vi "Autonomous Independent.vi"() -> ()   [LabVIEW 2016]
doc: "This VI is called when autonomous begins, and will automatically be terminated when autonomous ends. You can carry out timed or sensor driven robot movement independently without needing to return to the caller."
uses:
  <vilib>/Rock Robotics/WPI/Utilities/WPI_GetSetVariantRefNum.vi
  <vilib>/Rock Robotics/Network Tables/NT Read String.vi
  <vilib>/Rock Robotics/Network Tables/NT Write Numeric Array.vi
  <vilib>/Rock Robotics/WPI/RobotDrive/WPI_RobotDriveArcadeDrive_Standard(NoSaturation).vi
panel:
  in  "PID":T1
  out "Sensor2Pos":dbl
  out "Sensor1Pos":dbl
  in  "Rotational Target":dbl
  out "SensorPos 2":dbl
  out "SensorPos":dbl
  in  "Target":dbl
  out "Current Movement, for debugging":T2 {"Y Joystick Value" scale=1.0..-1.0; "X Joystick Value" scale=-1.0..1.0}
  in  "Array of robot movements":T3(array[cluster])=[{"X Joystick Value"=0.39393939393939403, "Y Joystick Value"=0.0, "Delay (sec)"=1.0, "Movement Name"="turn"}, {"X Joystick Value"=-0.3737373737373737, "Y Joystick Value"=0.0, "Delay (sec)"=1.0, "Movement Name"="turn back"}] {"Y Joystick Value" scale=1.0..-1.0; "X Joystick Value" scale=-1.0..1.0}
  # "Be sure to right-click and choose Data Operations>>Make Current Value default if you want to save the array values with the VI"
  # "Position Closed Loop"
  # "Positive=Clockwise"
  # "Rotate"
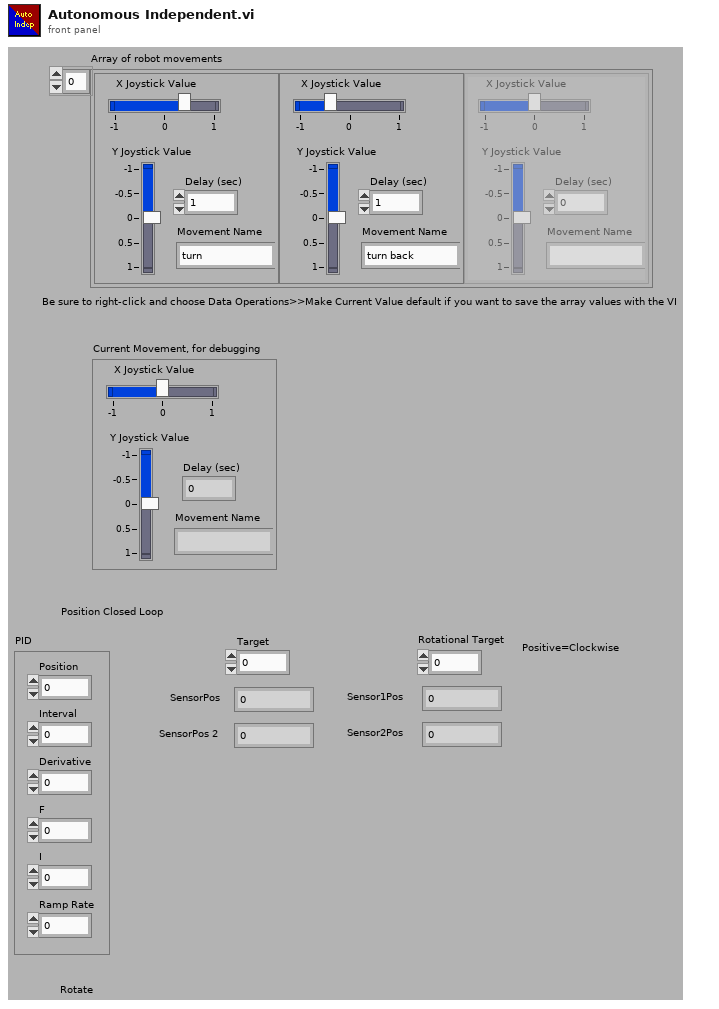
[diagram p1: front panel]
types:
  T1 = cluster{"Position":dbl, "Interval":dbl, "Derivative":dbl, "F":dbl, "I":dbl, "Ramp Rate":dbl}
  T2 = cluster{"X Joystick Value":dbl, "Y Joystick Value":dbl, "Delay (sec)":dbl, "Movement Name":string}
  T3 = cluster{"X Joystick Value":dbl, "Y Joystick Value":dbl, "Delay (sec)":dbl, "Movement Name":string}[]
  T4 = typedef "WPI_JoystickDevRef.ctl" = cluster{"Device":T5}
  T5 = typedef "WPI_JoystickDeviceEnum.ctl" = enum16{"USB 0", "USB 1", "USB 2", "USB 3", "USB 4", "USB 5"}
  T6 = typedef "WPI_RobotDriveDevRef.ctl" = cluster{"DevStatus":errorcluster, "Motors[]":T7[], "Square Inputs":bool, "Max Output":dbl}
  T7 = typedef "WPI_MotorControlDeviceRef.ctl" = cluster{"DeviceStatus":errorcluster, "Type":T8, "PWM":cluster{"PWM Channel":T9, "DeadBand":T10}, "CAN":cluster{"Device Number":u8, "SetOutput VI Ref":variant, "GetOutput VI Ref":variant, "Enable VI Ref":variant, "Disable VI Ref":variant, "Data":variant}, "Invert":bool}
  T8 = typedef "WPI_MotorControlType.ctl" = enum16{"PWM", "CAN"}
  T9 = typedef "FPGA_DIOPWMChannel.ctl" = enum8{"PWM 0", "PWM 1", "PWM 2", "PWM 3", "PWM 4", "PWM 5", "PWM 6", "PWM 7", "PWM 8", "PWM 9", "PWM MXP 0", "PWM MXP 1", "PWM MXP 2", "PWM MXP 3", "PWM MXP 4", "PWM MXP 5", "PWM MXP 6", "PWM MXP 7", "PWM MXP 8", "PWM MXP 9", "Invalid"}
  T10 = typedef "WPI_PWMDeadband.ctl" = cluster{"Name":string, "maxPositivePwm":i32, "minPositivePwm":i32, "centerPwm":i32, "maxNegativePwm":i32, "minNegativePwm":i32, "angularRange":u16}
  T11 = typedef "WPI_CANTalonSRX_GlobalStatus.ctl" = cluster{"Applied Throttle":dbl, "Module Enabled":bool, "CAN Error":errorcluster, "Closed Loop Error":dbl, "Forward Limit Switch Closed":bool, "Reverse Limit Switch Closed":bool, "Sensor Position":dbl, "Sensor Velocity":dbl, "Current":dbl, "Sticky Fault - Over Temp":bool, "Sticky Fault - Under Voltage":bool, "Sticky Fault - Forward Limit":bool, "Sticky Fault - Reverse Limit":bool, "Sticky Fault - Forward Soft Limit":bool, "Sticky Fault - Reverse Soft Limit":bool, "Brake is Enabled":bool, "Encoder Position":dbl, "Encoder Velocity":dbl, "Encoder Index Count":dbl, "Encoder A Pin State":bool, "Encoder B Pin State":bool, "Encoder Index Pin State":bool, "Analog In":dbl, "Analog In Velocity":dbl, "Temperature (C)":dbl, "Battery Voltage":dbl, "Control 5 Is Supported":bool, "Current Profile Slot Select":dbl, "Pos Div 8":bool, "Vel Div 4":bool, "Pulse Width Position":i32, "Pulse Width Velocity":i32, "Pulse Width Rise To Rise (us)":i32, "Pulse Width Rise To Fall (us)":i32, "Mot Prof Active Is Under Run":bool, "Mot Prof Active Has Under Run":bool, "Mot Prof Active Is Last":bool, "Mot Prof Active Velocity Only":bool, "Mot Prof Active Is Valid":bool, "Mot Prof Buffer Is Full":bool, "Mot Prof Active Profile Slot Select":i32, "Mot Prof NextID":i32, "Mot Prof Count":i32, "Mot Prof Active Velocity":dbl, "Mot Prof Active Position":dbl, "Mot Prof Output Enable":i32}
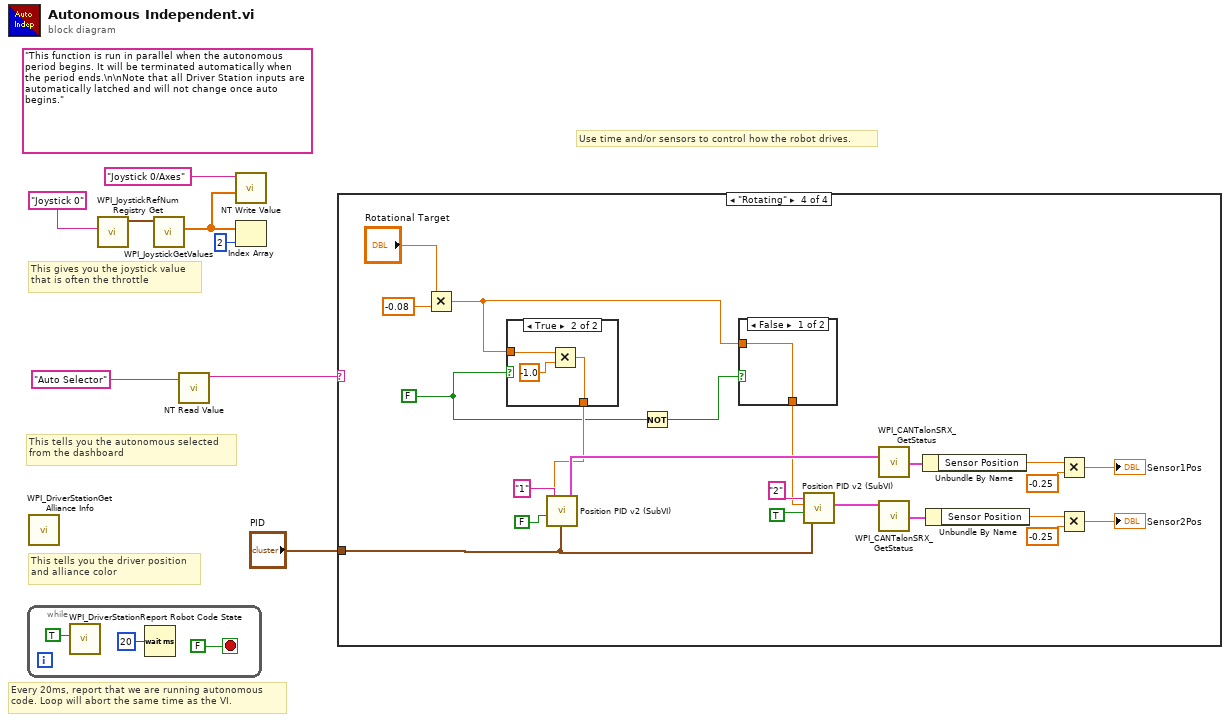
[diagram p0: block diagram]
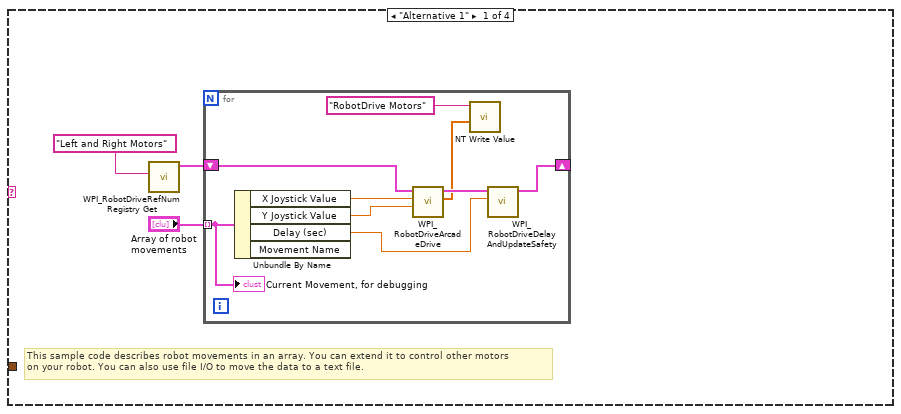
[diagram p2: hidden frame]
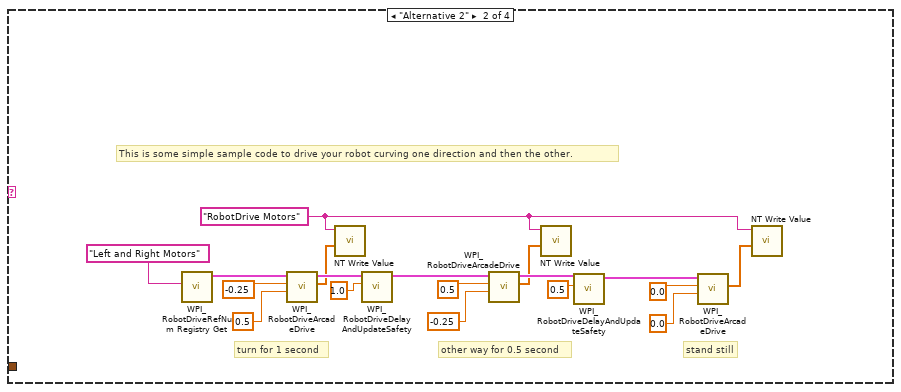
[diagram p3: hidden frame]
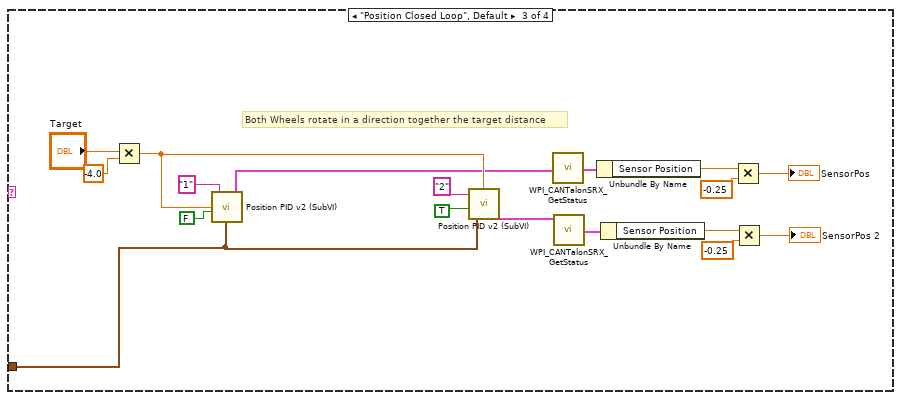
[diagram p4: hidden frame]
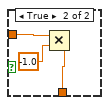
[diagram p5: hidden frame]
diagram:
  (unwired) "This function is run in parallel when the autonomous period begins. It will be terminated automatically when the period ends.\n\nNote that all Driver Station inputs are automatically latched and will not change once auto begins."
  # "This tells you the autonomous selected\nfrom the dashboard"
  # "Every 20ms, report that we are running autonomous\ncode. Loop will abort the same time as the VI."
  # "This gives you the joystick value\nthat is often the throttle"
  # "Use time and/or sensors to control how the robot drives."
  # "This tells you the driver position\nand alliance color"
  n1 = while {
    stop <- FALSE stop-if-true
    n2 = call <vilib>:"WPI_DriverStationReport Robot Code State.vi"("Autonomous"=TRUE) -> ()  [unwired: 10 in, 1 out]
    n3 = Wait (ms)(milliseconds to wait=u32 20) -> ()  [unwired: 1 out]
  }
  n4 = call <vilib>:"WPI_DriverStationGet Alliance Info.vi"() -> ()  [unwired: 12 out]
  n5 = call <vilib>:"WPI_JoystickRefNum Registry Get.vi"("refnum name"="Joystick 0") -> ("JoystickDevRef"=w7:T4)  [unwired: 1 in, 9 out]
  n6 = call <vilib>:"WPI_JoystickGetValues.vi"("JoystickDevRef"=w7) -> ("Axes"=w3:dbl[])  [unwired: 6 in, 4 out]
  n7 = call-poly <vilib>:"NT Read Value.vi"("Name"="Auto Selector") -> ("String"=w4:string)  [unwired: 9 in, 1 out]
  n8 = call-poly <vilib>:"NT Write Value.vi"("Numeric Array"=w3, "Name"="Joystick 0/Axes") -> ()  [unwired: 9 in, 1 out]
  n9 = Index Array(array=w3, index=2) -> ()  [unwired: 1 out]
  n10 = case shown="\"Rotating\"" w4 {
    tunnel: "PID" -> [_ _ w42 w62]
    frame "Alternative 1" {
      # "This sample code describes robot movements in an array. You can extend it to control other motors\non your robot. You can also use file I/O to move the data to a text file."
      n11 = call <vilib>:"WPI_RobotDriveRefNum Registry Get.vi"("refnum name"="Left and Right Motors") -> ("RobotDriveDevRef"=w13:T6)  [unwired: 1 in, 9 out]
      n12 = for {
        shift-right: [w21] -> _
        shift-left: w13 -> [w22]
        tunnel: "Array of robot movements" -> [w17] mode=indexing
        n13 = Unbundle By Name(w17) -> ("X Joystick Value"=w20:dbl, "Y Joystick Value"=w19:dbl, "Delay (sec)"=w18:dbl)  [unwired: 1 out]
        n14 = call-poly <vilib>:"WPI_RobotDriveArcadeDrive.vi"("Y axis value"=w19, "X axis value"=w20, "RobotDriveDevRef"=w22) -> ("Motor Values"=w15:dbl[], "RobotDriveDevRef"=w23:T6)  [unwired: 1 in, 6 out]
        n15 = call-poly <vilib>:"NT Write Value.vi"("Numeric Array"=w15, "Name"="RobotDrive Motors") -> ()  [unwired: 9 in, 1 out]
        n16 = call <vilib>:"WPI_RobotDriveDelayAndUpdateSafety.vi"("Delay (s)"=w18, "RobotDriveDevRef"=w23) -> ("RobotDriveDevRef 2"=w21:T6)  [unwired: 8 in, 1 out]
        "Current Movement, for debugging" <- w17
      }
    }
    frame "Alternative 2" {
      w25 = "RobotDrive Motors" ("Name")
      # "This is some simple sample code to drive your robot curving one direction and then the other."
      # "stand still"
      # "other way for 0.5 second"
      # "turn for 1 second"
      n17 = call <vilib>:"WPI_RobotDriveRefNum Registry Get.vi"("refnum name"="Left and Right Motors") -> ("RobotDriveDevRef"=w41:T6)  [unwired: 1 in, 9 out]
      n18 = call-poly <vilib>:"WPI_RobotDriveArcadeDrive.vi"("Y axis value"=0.5 ("X axis value"), "X axis value"=-0.25, "RobotDriveDevRef"=w41) -> ("Motor Values"=w24:dbl[], "RobotDriveDevRef"=w34:T6)  [unwired: 1 in, 6 out]
      n19 = call-poly <vilib>:"NT Write Value.vi"("Numeric Array"=w24, "Name"=w25) -> ()  [unwired: 9 in, 1 out]
      n20 = call <vilib>:"WPI_RobotDriveDelayAndUpdateSafety.vi"("Delay (s)"=1.0, "RobotDriveDevRef"=w34) -> ("RobotDriveDevRef 2"=w35:T6)  [unwired: 8 in, 1 out]
      n21 = call-poly <vilib>:"WPI_RobotDriveArcadeDrive.vi"("Y axis value"=-0.25 ("X axis value"), "X axis value"=0.5, "RobotDriveDevRef"=w35) -> ("Motor Values"=w26:dbl[], "RobotDriveDevRef"=w36:T6)  [unwired: 1 in, 6 out]
      n22 = call-poly <vilib>:"NT Write Value.vi"("Numeric Array"=w26, "Name"=w25) -> ()  [unwired: 9 in, 1 out]
      n23 = call <vilib>:"WPI_RobotDriveDelayAndUpdateSafety.vi"("Delay (s)"=0.5, "RobotDriveDevRef"=w36) -> ("RobotDriveDevRef 2"=w37:T6)  [unwired: 8 in, 1 out]
      n24 = call-poly <vilib>:"WPI_RobotDriveArcadeDrive.vi"("Y axis value"=0.0 ("X axis value"), "X axis value"=0.0, "RobotDriveDevRef"=w37) -> ("Motor Values"=w27:dbl[])  [unwired: 1 in, 7 out]
      n25 = call-poly <vilib>:"NT Write Value.vi"("Numeric Array"=w27, "Name"=w25) -> ()  [unwired: 9 in, 1 out]
    }
    frame "Position Closed Loop", Default {
      # "Both Wheels rotate in a direction together the target distance"
      n26 = Multiply(x="Target", y=-4.0) -> (x*y=w53:dbl)
      n27 = call "Position PID v2 (SubVI).vi"("Cluster"=w42, "Reverse Feedback"=FALSE, "Target"=w53, "Motor Refnum"="1" ("Motor Ref Num")) -> ("CAN Talon SRX Ref"=w43:T7)
      n28 = call "Position PID v2 (SubVI).vi"("Cluster"=w42, "Reverse Feedback"=TRUE, "Target"=w53, "Motor Refnum"="2" ("Motor Ref Num")) -> ("CAN Talon SRX Ref"=w44:T7)
      n29 = call <vilib>:"WPI_CANTalonSRX_GetStatus.vi"("CAN Talon SRX Ref"=w43) -> ("Talon SRX Status"=w56:T11)  [unwired: 8 in, 2 out]
      n30 = call <vilib>:"WPI_CANTalonSRX_GetStatus.vi"("CAN Talon SRX Ref"=w44) -> ("Talon SRX Status"=w46:T11)  [unwired: 8 in, 2 out]
      n31 = Unbundle By Name(w56) -> ("Sensor Position"=w55:dbl)
      n32 = Unbundle By Name(w46) -> ("Sensor Position"=w47:dbl)
      n33 = Multiply(x=w55, y=-0.25) -> (x*y=→"SensorPos":dbl)
      n34 = Multiply(x=w47, y=-0.25) -> (x*y=→"SensorPos 2":dbl)
    }
    frame "Rotating" {
      w61 = FALSE
      n35 = Multiply(x="Rotational Target", y=-0.08) -> (x*y=w66:dbl)
      n36 = case shown="True" w61 {
        tunnel: w66 -> [w86 w89]
        tunnel: [w86 w88] -> w64
        frame False {
        }
        frame True {
          n37 = Multiply(x=w89, y=-1.0) -> (x*y=w88:dbl)
        }
      }
      n38 = call "Position PID v2 (SubVI).vi"("Cluster"=w62, "Reverse Feedback"=FALSE, "Target"=w64, "Motor Refnum"="1" ("Motor Ref Num")) -> ("CAN Talon SRX Ref"=w67:T7)
      n39 = Not(x=w61) -> (.not. x?=w63:bool)
      n40 = case shown="False" w63 {
        tunnel: w66 -> [w82 w85]
        tunnel: [w82 w84] -> w65
        frame False {
        }
        frame True {
          n41 = Multiply(x=w85, y=-1.0) -> (x*y=w84:dbl)
        }
      }
      n42 = call "Position PID v2 (SubVI).vi"("Cluster"=w62, "Reverse Feedback"=TRUE, "Target"=w65, "Motor Refnum"="2" ("Motor Ref Num")) -> ("CAN Talon SRX Ref"=w68:T7)
      n43 = call <vilib>:"WPI_CANTalonSRX_GetStatus.vi"("CAN Talon SRX Ref"=w67) -> ("Talon SRX Status"=w78:T11)  [unwired: 8 in, 2 out]
      n44 = call <vilib>:"WPI_CANTalonSRX_GetStatus.vi"("CAN Talon SRX Ref"=w68) -> ("Talon SRX Status"=w70:T11)  [unwired: 8 in, 2 out]
      n45 = Unbundle By Name(w78) -> ("Sensor Position"=w77:dbl)
      n46 = Unbundle By Name(w70) -> ("Sensor Position"=w71:dbl)
      n47 = Multiply(x=w77, y=-0.25) -> (x*y=→"Sensor1Pos":dbl)
      n48 = Multiply(x=w71, y=-0.25) -> (x*y=→"Sensor2Pos":dbl)
    }
  }
